vi "Dequeuer.vi"() -> ()   [LabVIEW 2020]
panel:
  out "Waveform Chart":dbl(graph)
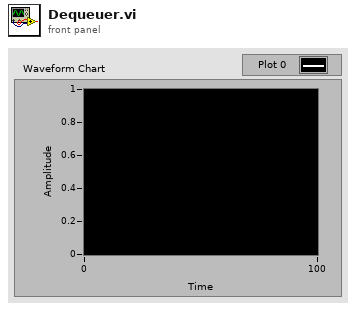
[diagram p1: front panel]
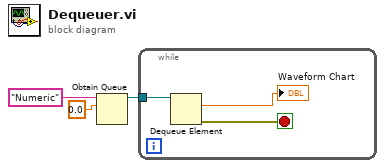
[diagram p0: block diagram]
diagram:
  n1 = Obtain Queue(name (unnamed)="Numeric", element data type=0.0) -> (queue out=w1:refnum<queue>)  [unwired: 3 in, 2 out]
  n2 = while {
    tunnel: w1 -> [w6]
    stop <- w4 stop-if-true
    n3 = Dequeue Element(queue=w6) -> (element=→"Waveform Chart":dbl, error out=w4:errorcluster)  [unwired: 2 in, 2 out]
  }
